vi "Configure Power Analysis (Harmonics).vi"(8 "error in (no error)":errorcluster, 9 "Standard (0: IEC 61000- 3- 2 Class A)":i32(ring) items=["IEC 61000- 3- 2 Class A", "IEC 61000- 3- 2 Class B", "IEC 61000- 3- 2 Class C", "IEC 61000- 3- 2 Class D"], 10 "Line Frequency (0: 50 Hz)":i32(ring) items=["50 Hz", "60 Hz", "400 Hz"], 11 "VISA resource name":refnum<visa-resource-name>) -> (0 "error out":errorcluster, 3 "VISA resource name out":refnum<visa-resource-name>)   [LabVIEW 2010, in "Agilent 2000 3000 X-Series.lvlib"]
doc: "Applies the current harmonics analysis.\n\n<B>Note(s):</B>\nSwitching power supplies draw a range of harmonics from the AC mains.\n\nStandard limits are set for these harmonics because these harmonics can travel back to the supply grid and cause problems with other devices on the grid.\n\nUse the Current Harmonics analysis to test a switching power supply's current harmonics to pre-compliance standard of IEC61000- 3- 2 (Class A, B, C, or D). The analysis presents up to 40 harmonics.\n\nUse <B>Read Measurement (Harmonics Power Analysis).vi</B> to read the result of this power analysis."
uses:
  <instrlib>/Agilent 2000 3000 X-Series/Agilent 2000 3000 X-Series.lvlib
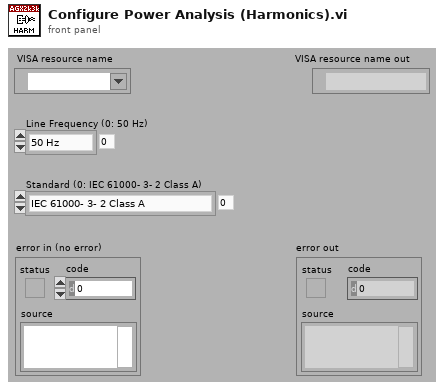
[diagram p1: front panel]
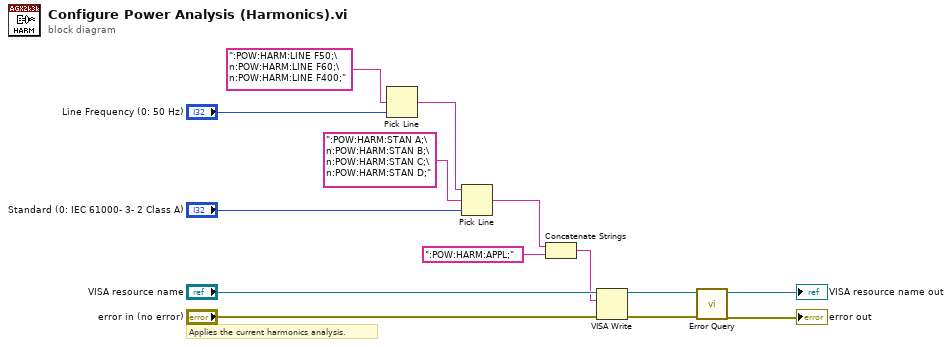
[diagram p0: block diagram]
diagram:
  # "Applies the current harmonics analysis."
  n1 = Pick Line(multi-line string=":POW:HARM:LINE F50;\n:POW:HARM:LINE F60;\n:POW:HARM:LINE F400;", line index="Line Frequency (0: 50 Hz)") -> (output string=w10:string)  [unwired: 1 out]
  n2 = Pick Line(string ("")=w10, multi-line string=":POW:HARM:STAN A;\n:POW:HARM:STAN B;\n:POW:HARM:STAN C;\n:POW:HARM:STAN D;", line index="Standard (0: IEC 61000- 3- 2 Class A)") -> (output string=w3:string)
  n3 = Concatenate Strings(w3, ":POW:HARM:APPL;") -> (w1:string)
  n4 = VISA Write(VISA resource name="VISA resource name", write buffer=w1, error in (no error)="error in (no error)") -> (VISA resource name out=w7:refnum<visa-resource-name>, error out=w6:errorcluster)  [unwired: 1 out]
  n5 = call <instrlib>:"Error Query.vi"("error in (no error)"=w6, "VISA resource name"=w7) -> ("error out"=→"error out":errorcluster, "VISA resource name out"=→"VISA resource name out":refnum<visa-resource-name>)  [unwired: 8 out]
